vi "Host - Thrusters signal Update (SubVI).vi"(11 "Thruster Status":T1) -> (3 "Thrusters Signal":T2)   [LabVIEW 2021]
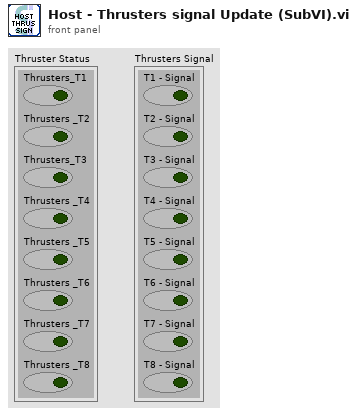
[diagram p1: front panel]
types:
  T1 = cluster{"Thrusters_T1":bool, "Thrusters _T2":bool, "Thrusters_T3":bool, "Thrusters _T4":bool, "Thrusters _T5":bool, "Thrusters _T6":bool, "Thrusters _T7":bool, "Thrusters _T8":bool}
  T2 = cluster{"T1 - Signal":bool, "T2 - Signal":bool, "T3 - Signal":bool, "T4 - Signal":bool, "T5 - Signal":bool, "T6 - Signal":bool, "T7 - Signal":bool, "T8 - Signal":bool}
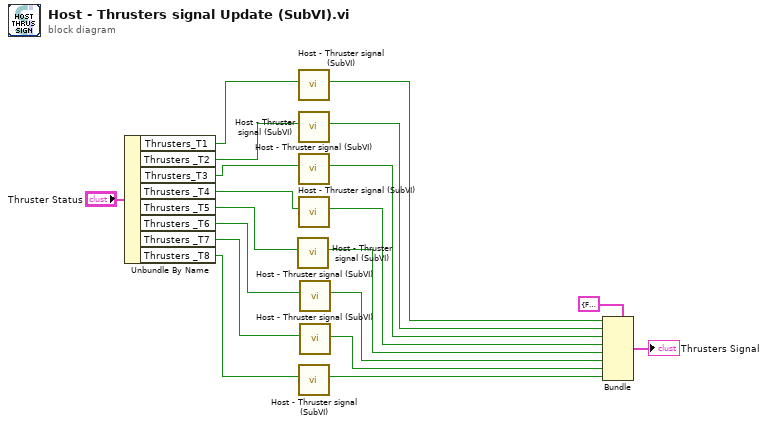
[diagram p0: block diagram]
diagram:
  n1 = Unbundle By Name("Thruster Status") -> ("Thrusters_T1"=w2:bool, "Thrusters _T2"=w3:bool, "Thrusters_T3"=w4:bool, "Thrusters _T4"=w5:bool, "Thrusters _T5"=w6:bool, "Thrusters _T6"=w7:bool, "Thrusters _T7"=w8:bool, "Thrusters _T8"=w9:bool)
  n2 = call "Host - Thruster signal (SubVI).vi"("T Status"=w6) -> ("T - Signal"=w14:bool)  [unwired: 10 in]
  n3 = call "Host - Thruster signal (SubVI).vi"("T Status"=w2) -> ("T - Signal"=w10:bool)  [unwired: 10 in]
  n4 = call "Host - Thruster signal (SubVI).vi"("T Status"=w3) -> ("T - Signal"=w11:bool)  [unwired: 10 in]
  n5 = call "Host - Thruster signal (SubVI).vi"("T Status"=w4) -> ("T - Signal"=w12:bool)  [unwired: 10 in]
  n6 = call "Host - Thruster signal (SubVI).vi"("T Status"=w5) -> ("T - Signal"=w13:bool)  [unwired: 10 in]
  n7 = call "Host - Thruster signal (SubVI).vi"("T Status"=w9) -> ("T - Signal"=w17:bool)  [unwired: 10 in]
  n8 = call "Host - Thruster signal (SubVI).vi"("T Status"=w7) -> ("T - Signal"=w15:bool)  [unwired: 10 in]
  n9 = call "Host - Thruster signal (SubVI).vi"("T Status"=w8) -> ("T - Signal"=w16:bool)  [unwired: 10 in]
  n10 = Bundle(cluster=T2 {"T1 - Signal"=FALSE, "T2 - Signal"=FALSE, "T3 - Signal"=FALSE, "T4 - Signal"=FALSE, "T5 - Signal"=FALSE, "T6 - Signal"=FALSE, "T7 - Signal"=FALSE, "T8 - Signal"=FALSE}, "T1 - Signal"=w10, "T2 - Signal"=w11, "T3 - Signal"=w12, "T4 - Signal"=w13, "T5 - Signal"=w14, "T6 - Signal"=w15, "T7 - Signal"=w16, "T8 - Signal"=w17) -> (→"Thrusters Signal":T2)
